vi "SESW Specific Enthalpy of Saline Water (J to Kg).vi"(1 "Salinity":dbl, 2 "Sailne Water Temprature":dbl[unit]) -> (0 "SESW":dbl[unit])   [LabVIEW 2018]
panel:
  out "Reduction Part":dbl[unit]
  out "SEPW":dbl[unit]
  out "Saline Water Temprature":dbl[unit](slide) scale=0.0..100.0
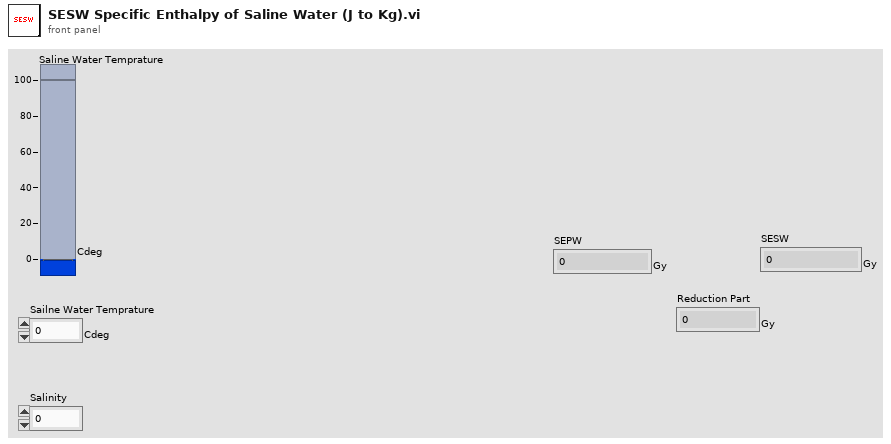
[diagram p1: front panel]
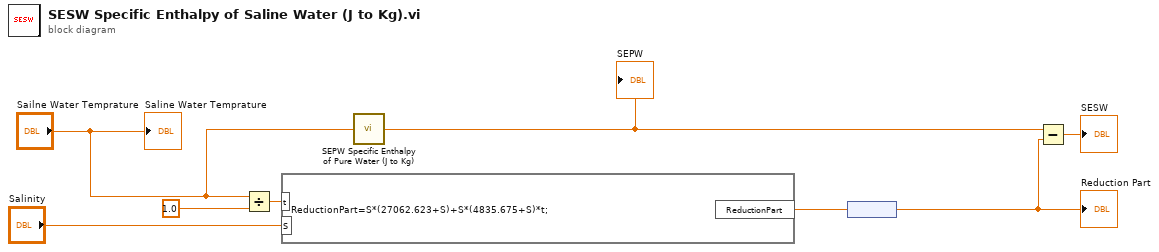
[diagram p0: block diagram]
diagram:
  n1 = Divide(x="Sailne Water Temprature", y=dbl[unit] 1.0) -> (x/y=w8:dbl)
  n2 = formula code="ReductionPart=S*(27062.623+S)+S*(4835.675+S)*t;"("t"=w8, "S"="Salinity") -> ("ReductionPart"=w6:dbl)
  n3 = call "SEPW Specific Enthalpy of Pure Water (J to Kg).vi"("Temp Pure Wate"="Sailne Water Temprature") -> ("SEPW"=w2:dbl[unit])
  "SEPW" <- w2
  n4 = node(w6) -> (w5:dbl[unit])
  "Reduction Part" <- w5
  n5 = Subtract(x=w2, y=w5) -> (x-y=→"SESW":dbl[unit])
  "Saline Water Temprature" <- "Sailne Water Temprature"
